vi "Spin Image.vi"(9 "Angle [rad]":dbl, 10 "RotationPoint":cluster{"x":i16, "y":i16}, 11 "Image In":T1) -> (3 "Image Out":T1)   [LabVIEW 2017, in "ONNX Angle Class Library.lvlib"]
doc: "Created IvanLis by LabVIEW Portal\nProfile: http://labviewportal.org/memberlist.php?mode=viewprofile&u=987\neMail: IvanLisanov@gMail.com\nTelegram: https://t.me/IvanLis"
uses:
  ONNX Angle Class Library.lvlib
  <vilib>/picture/picture.llb/imagedata.ctl
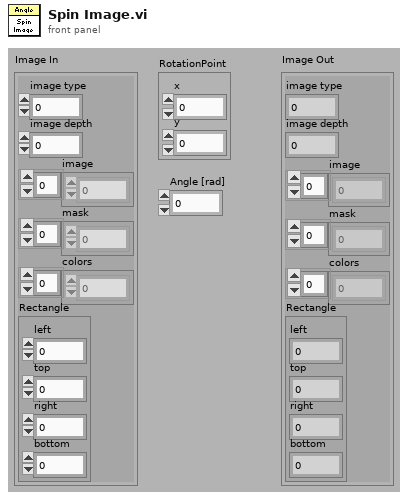
[diagram p1: front panel]
types:
  T1 = typedef "imagedata.ctl" = cluster{"image type":i32, "image depth":i32, "image":u8[], "mask":u8[], "colors":u32[], "Rectangle":cluster{"left":i16, "top":i16, "right":i16, "bottom":i16}}
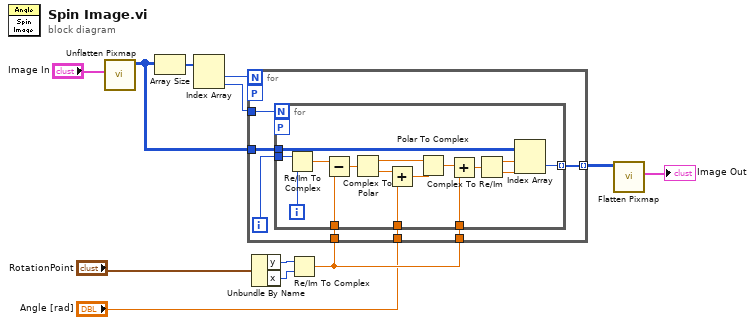
[diagram p0: block diagram]
diagram:
  n1 = call <vilib>:"Unflatten Pixmap.vi"("image data"="Image In") -> ("24-bit pixmap"=w6:u32[][])  [unwired: 4 in, 6 out]
  n2 = Array Size(array=w6) -> (size(s)=w2:i32[])
  n3 = Index Array(array=w2) -> (element #1=w10:i32, element #2=w11:i32)  [unwired: 2 in]
  n4 = Unbundle By Name("RotationPoint") -> ("y"=w8:i16, "x"=w9:i16)
  n5 = Re/Im To Complex(1:w9, 2:w8) -> (0:w12:cdb)
  n6 = for {
    N: w10 -> [_]
    tunnel: "Angle [rad]" -> [w19]
    tunnel: w6 -> [w18]
    tunnel: w12 -> [w17]
    tunnel: [w16] -> w5 mode=indexing
    tunnel: w11 -> [w15]
    tunnel: w12 -> [w13]
    workers-P: _ -> [_]
    i -> [w14]
    n7 = for {
      N: w15 -> [_]
      tunnel: w18 -> [w29]
      tunnel: w19 -> [w32]
      tunnel: w17 -> [w26]
      tunnel: [w25] -> w16 mode=indexing
      tunnel: w14 -> [w23]
      tunnel: w13 -> [w21]
      workers-P: _ -> [_]
      i -> [w24]
      n8 = Re/Im To Complex(1:w24, 2:w23) -> (0:w22:cdb)
      n9 = Subtract(x=w22, y=w21) -> (x-y=w20:cdb)
      n10 = Complex To Polar(r * e^(i*theta)=w20) -> (r=w35:dbl, theta=w34:dbl)
      n11 = Add(x=w34, y=w32) -> (x+y=w33:dbl)
      n12 = Polar To Complex(1:w33, 2:w35) -> (0:w31:cdb)
      n13 = Add(x=w31, y=w26) -> (x+y=w27:cdb)
      n14 = Complex To Re/Im(x + iy=w27) -> (x=w30:dbl, y=w28:dbl)
      n15 = Index Array(array=w29, index (row)=w30, index (col)=w28) -> (element=w25:u32)
    }
  }
  n16 = call <vilib>:"Flatten Pixmap.vi"("24-bit pixmap"=w5) -> ("image data"=→"Image Out":T1)  [unwired: 10 in]
